vi "DAQmx Read Strain (SubVI).vi"(0 "cDAQ Chassis":i32=2, 5 "9237 (A) Slot":i32=1, 7 "9237 (B) Slot":i32=2, 9 "9237 (C) Slot":i32=2, 11 "Strain Config":T1={"Filter"={"Low-Pass Cut-Off [Hz]"=2.0, "HI/LO Trim [%]"=5.0, "Smooth Size"=3}, "Number of Samples"=6250, "Settings (A)"={"voltage excitation source"=10200, "bridge configuration"=10182, "voltage excitation value"=10.0, "use excitation for scaling"=TRUE, "MIN"=0.0, "MAX"=0.0}, "Settings (B)"={"voltage excitation source"=10200, "bridge configuration"=10182, "voltage excitation value"=10.0, "use excitation for scaling"=TRUE, "MIN"=0.0, "MAX"=0.0}, "Settings (C)"={"voltage excitation source"=10200, "bridge configuration"=10182, "voltage excitation value"=10.0, "use excitation for scaling"=TRUE, "MIN"=0.0, "MAX"=0.0}} {"Settings (C)"."voltage excitation source" items=["Internal"=10200, "External"=10167, "None"=10230]; "Settings (C)"."bridge configuration" items=["Full Bridge"=10182, "Half Bridge"=10187, "Quarter Bridge"=10270, "No Bridge"=10228]; "Settings (B)"."voltage excitation source" items=["Internal"=10200, "External"=10167, "None"=10230]; "Settings (B)"."bridge configuration" items=["Full Bridge"=10182, "Half Bridge"=10187, "Quarter Bridge"=10270, "No Bridge"=10228]; "Settings (A)"."voltage excitation source" items=["Internal"=10200, "External"=10167, "None"=10230]; "Settings (A)"."bridge configuration" items=["Full Bridge"=10182, "Half Bridge"=10187, "Quarter Bridge"=10270, "No Bridge"=10228]}, 12 "Stop Program":bool) -> (4 "Strain Task":refnum<k21>="Relay Control", 6 "(A) Strain":T2 {"Signals" format="%.2p"}, 8 "(B) Strain":T2, 10 "(C) Strain":T2, 13 "Ch0 Raw":dbl[](array[numeric]), 14 "Ch0 Filtered":dbl, 15 "Strain Error":errorcluster={"status"=TRUE, "code"=-200170, "source"="DAQmx Create Channel (DO-Digital Output).vi:1<append>\n<B>Task Name: </B>Relay Control"})   [LabVIEW 2010]
uses:
  <vilib>/Analysis/3filter.llb/Filter Passband Type.ctl
  <vilib>/DAQmx/read.llb/DAQmx Read (Analog 2D DBL NChan NSamp).vi
  <vilib>/daqmx/miscellaneous.llb/DAQmx Fill In Error Info.vi
  <vilib>/Analysis/3filter.llb/Butterworth Filter (DBL).vi
  <vilib>/DAQmx/configure/timing.llb/DAQmx Timing (Sample Clock).vi
  <vilib>/DAQmx/create/channels.llb/DAQmx Create Channel (AI-Voltage-Custom with Excitation).vi
  <vilib>/Analysis/NI_AALBase.lvlib
panel:
  in  "Error Input":errorcluster
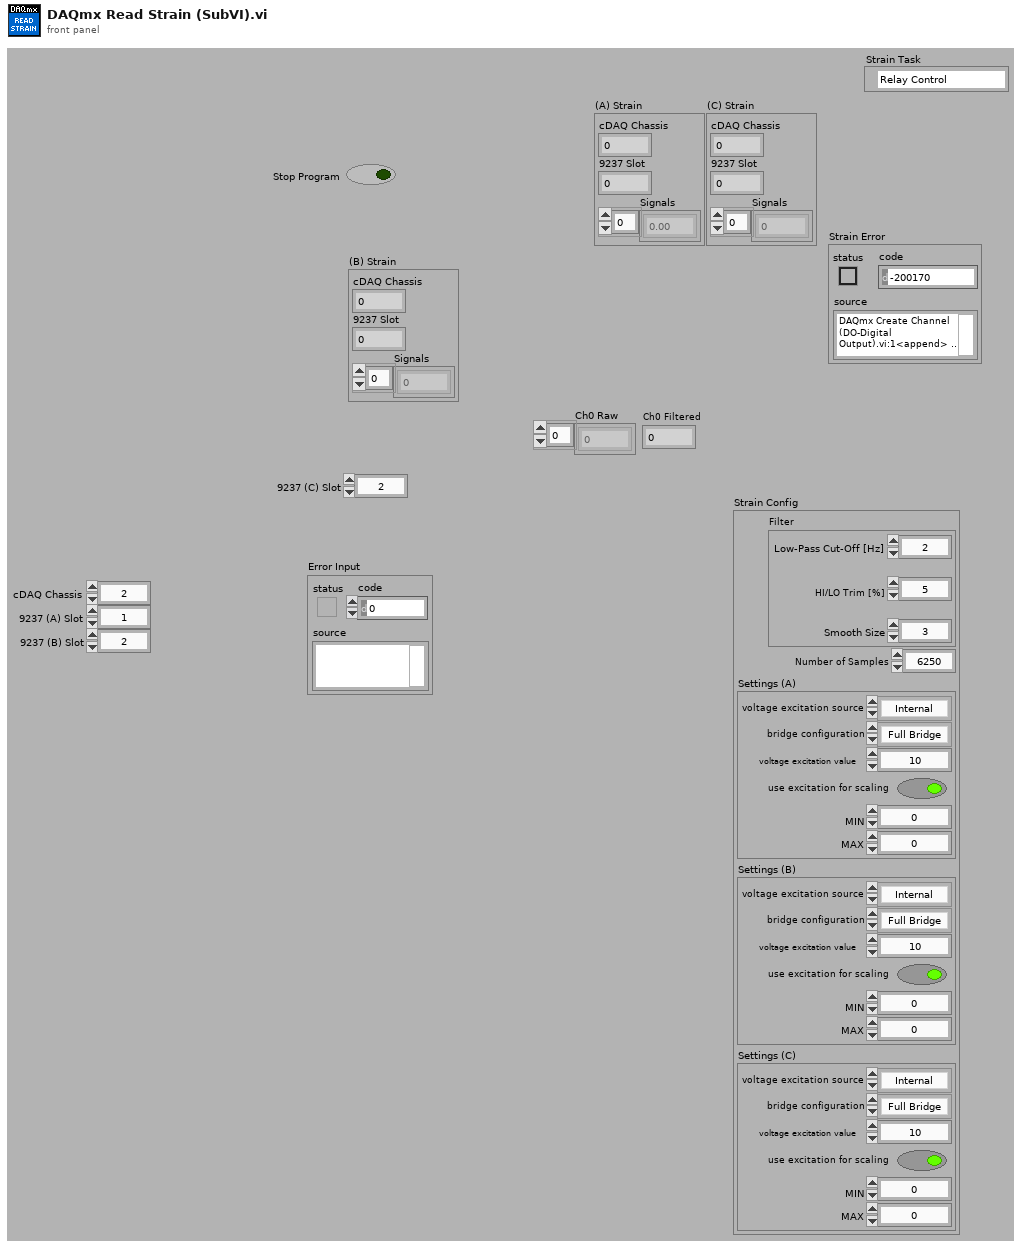
[diagram p1: front panel]
types:
  T1 = cluster{"Filter":cluster{"Low-Pass Cut-Off [Hz]":dbl, "HI/LO Trim [%]":dbl, "Smooth Size":i32}, "Number of Samples":i32, "Settings (A)":cluster{"voltage excitation source":i32, "bridge configuration":i32, "voltage excitation value":dbl, "use excitation for scaling":bool, "MIN":dbl, "MAX":dbl}, "Settings (B)":cluster{"voltage excitation source":i32, "bridge configuration":i32, "voltage excitation value":dbl, "use excitation for scaling":bool, "MIN":dbl, "MAX":dbl}, "Settings (C)":cluster{"voltage excitation source":i32, "bridge configuration":i32, "voltage excitation value":dbl, "use excitation for scaling":bool, "MIN":dbl, "MAX":dbl}}
  T2 = cluster{"cDAQ Chassis":i32, "9237 Slot":i32, "Signals":dbl[]}
  T3 = typedef "NI_AALBase.lvlib/Filter Passband Type.ctl" = enum32{"Lowpass", "Highpass", "Bandpass", "Bandstop"}
  T4 = cluster{"Low-Pass Cut-Off [Hz]":dbl, "HI/LO Trim [%]":dbl, "Smooth Size":i32}
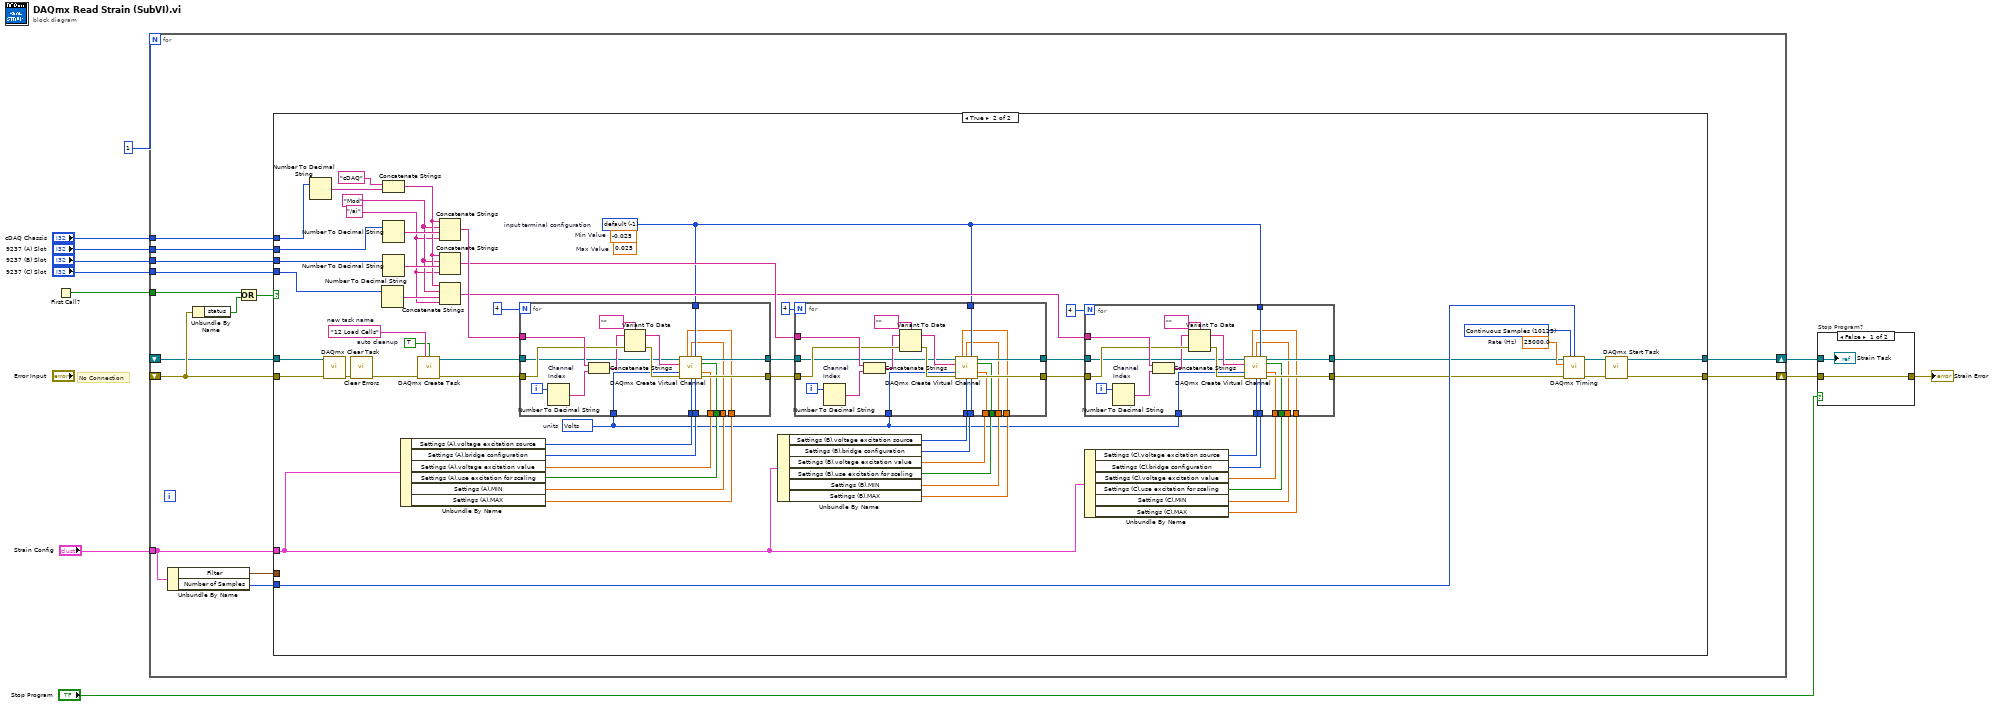
[diagram p0: block diagram]
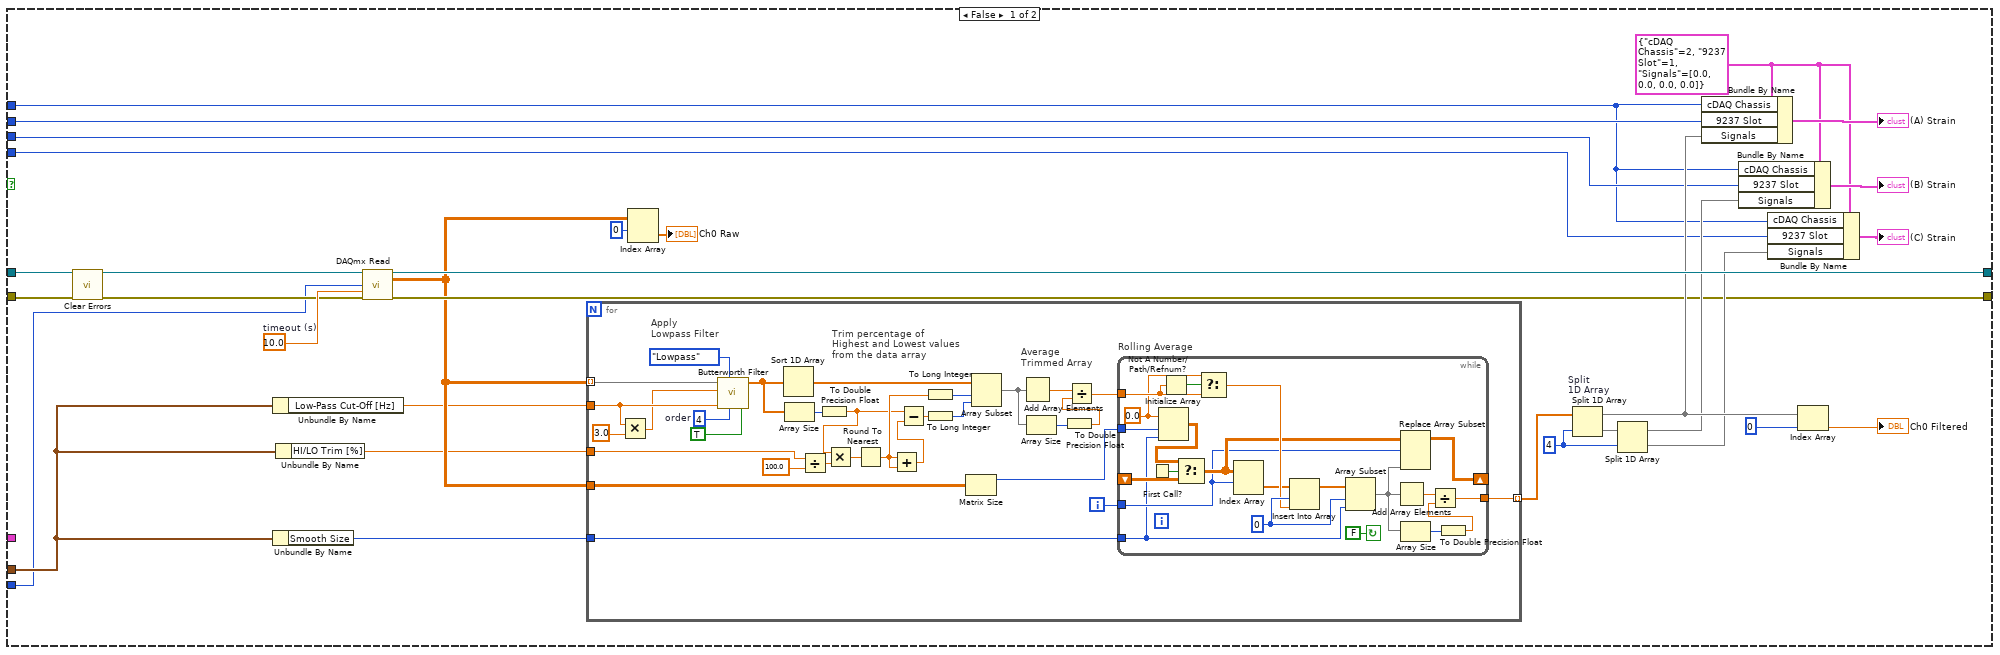
[diagram p2: hidden frame]
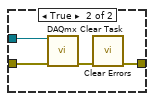
[diagram p3: hidden frame]
diagram:
  # "No Connection"
  n1 = First Call?() -> (First Call?: T/F=w7:bool)
  n2 = for {
    N: 1 -> [_]
    tunnel: "9237 (A) Slot" -> [w25]
    tunnel: "9237 (B) Slot" -> [w24]
    tunnel: "9237 (C) Slot" -> [w23]
    tunnel: "cDAQ Chassis" -> [w22]
    tunnel: w7 -> [w20]
    shift-right: [w18] -> w2
    shift-left: _ -> [w17]
    shift-right: [w16] -> w3
    shift-left: _ -> [w21]
    tunnel: "Strain Config" -> [w12]
    n3 = Unbundle By Name(w12) -> ("Filter"=w14:T4, "Number of Samples"=w13:i32)
    n4 = Unbundle By Name(w21) -> ("status"=w19:bool)
    n5 = Or(x=w20, y=w19) -> (x .or. y?=w15:bool)
    n6 = case shown="True" w15 {
      tunnel: w21 -> [w55 w151]
      tunnel: [w32 w154] -> w16
      tunnel: [w45 w153] -> w18
      tunnel: w17 -> [w46 w152]
      tunnel: w22 -> [w36 w150]
      tunnel: w25 -> [w44 w149]
      tunnel: w24 -> [w40 w148]
      tunnel: w23 -> [w35 w145]
      tunnel: w14 -> [w28 _]
      tunnel: w13 -> [w26 w138]
      tunnel: w12 -> [_ w133]
      frame False {
        w37 = T2 {"cDAQ Chassis"=2, "9237 Slot"=1, "Signals"=[0.0, 0.0, 0.0, 0.0]}
        w49 = 4 ("index")
        w47 = 10.0  # timeout (s)
        n7 = call <vilib>:"Clear Errors.vi"("error in (no error)"=w55) -> ("error out"=w33:errorcluster)  [unwired: 6 in]
        n8 = Unbundle By Name(w28) -> ("Low-Pass Cut-Off [Hz]"=w30:dbl)
        n9 = Unbundle By Name(w28) -> ("Smooth Size"=w27:i32)
        n10 = Unbundle By Name(w28) -> ("HI/LO Trim [%]"=w29:dbl)
        n11 = call-poly <vilib>:"DAQmx Read.vi"("task/channels in"=w46, "number of samples per channel"=w26, "timeout"=w47, "error in"=w33) -> ("task out"=w45:refnum<k21>, "data"=w31:dbl[][], "error out"=w32:errorcluster)  [unwired: 9 in]
        n12 = for {
          tunnel: w31 -> [w82] mode=indexing
          tunnel: [w57] -> w52 mode=indexing
          tunnel: w30 -> [w83]
          tunnel: w31 -> [w60]
          tunnel: w27 -> [w58]
          tunnel: w29 -> [w56]
          i -> [w61]
          w81 = 4  # order
          # "Average\nTrimmed Array"
          # "Trim percentage of\nHighest and Lowest values\nfrom the data array"
          # "Apply \nLowpass Filter"
          n13 = Multiply(x=w83, y=3.0) -> (x*y=w77:dbl)
          n14 = call-poly <vilib>:"Butterworth Filter.vi"("init/cont (init:F)"=TRUE, "order"=w81, "filter type"=Filter_Passband_Type."Lowpass", "low cutoff freq: fl"=w83, "sampling freq: fs"=w77, "X"=w82) -> ("Filtered X"=w85:dbl[])  [unwired: 2 in, 1 out]
          n15 = Sort 1D Array(array=w85) -> (sorted array=w70:dbl[])
          n16 = Array Size(array=w85) -> (size(s)=w76:i32)
          n17 = Divide(x=w56, y=100.0) -> (x/y=w66:dbl)
          n18 = To Double Precision Float(number=w76) -> (double precision float=w68:dbl)
          n19 = Multiply(x=w68, y=w66) -> (x*y=w74:dbl)
          n20 = Round To Nearest(number=w74) -> (nearest integer value=w73:dbl)
          n21 = Add(x=w73, y=w73) -> (x+y=w69:dbl)
          n22 = Subtract(x=w68, y=w69) -> (x-y=w75:dbl)
          n23 = To Long Integer(number=w73) -> (32bit integer=w71:i32)
          n24 = To Long Integer(number=w75) -> (32bit integer=w72:i32)
          n25 = Matrix Size(0:w60) -> (1:w59:i32)  [unwired: 1 out]
          n26 = Array Subset(array=w70, index=w71, length=w72) -> (w84:dbl[])
          n27 = Add Array Elements(numeric array=w84) -> (sum=w64:dbl)
          n28 = Array Size(array=w84) -> (size(s)=w65:i32)
          n29 = To Double Precision Float(number=w65) -> (double precision float=w63:dbl)
          n30 = Divide(x=w64, y=w63) -> (x/y=w62:dbl)
          n31 = while "Rolling Average" {
            tunnel: w62 -> [w104]
            tunnel: w58 -> [w88]
            shift-right: [w94] -> _
            shift-left: _ -> [w92]
            tunnel: [w105] -> w57
            tunnel: w61 -> [w90]
            tunnel: w59 -> [w87]
            stop <- FALSE continue-if-true
            w97 = 0.0
            w102 = 0
            n32 = First Call?() -> (First Call?: T/F=w99:bool)
            n33 = Initialize Array(w97, w87, w88) -> (w89:dbl[][])
            n34 = Not A Number/Path/Refnum?(number/path/refnum=w104) -> (NaN/Path/Refnum?=w98:bool)
            n35 = Select(t=w89, s=w99, f=w92) -> (s? t:f=w91:dbl[][])
            n36 = Select(t=w97, s=w98, f=w104) -> (s? t:f=w96:dbl)
            n37 = Index Array(array=w91, index (row)=w90) -> (element=w93:dbl[])  [unwired: 1 in]
            n38 = Insert Into Array(array=w93, index=w102, new element=w96) -> (w103:dbl[])
            n39 = Array Subset(array=w103, index=w102, length=w88) -> (w95:dbl[])
            n40 = Add Array Elements(numeric array=w95) -> (sum=w101:dbl)
            n41 = Replace Array Subset(array=w91, new element=w95, index (row)=w90) -> (w94:dbl[][])  [unwired: 1 in]
            n42 = Array Size(array=w95) -> (size(s)=w100:i32)
            n43 = To Double Precision Float(number=w100) -> (double precision float=w86:dbl)
            n44 = Divide(x=w101, y=w86) -> (x/y=w105:dbl)
          }
        }
        n45 = Index Array(array=w31, index (row)=0) -> (element=→"Ch0 Raw":dbl[])  [unwired: 1 in]
        n46 = Split 1D Array "Split\n1D Array"(array=w52, index=w49) -> (first subarray=w43:dbl[], second subarray=w48:dbl[])
        n47 = Split 1D Array(array=w48, index=w49) -> (first subarray=w39:dbl[], second subarray=w34:dbl[])
        n48 = Bundle By Name(cluster=w37, "cDAQ Chassis"=w36, "9237 Slot"=w44, "Signals"=w43) -> (→"(A) Strain":T2)
        n49 = Bundle By Name(cluster=w37, "cDAQ Chassis"=w36, "9237 Slot"=w40, "Signals"=w39) -> (→"(B) Strain":T2)
        n50 = Bundle By Name(cluster=w37, "cDAQ Chassis"=w36, "9237 Slot"=w35, "Signals"=w34) -> (→"(C) Strain":T2)
        n51 = Index Array(array=w43, index=0) -> (element=→"Ch0 Filtered":dbl)
      }
      frame True {
        (unwired) 0.025  # Max Value
        (unwired) -0.025  # Min Value
        w139 = 25000.0  # Rate (Hz)
        w140 = 10123 items=["Finite Samples"=10178, "Continuous Samples"=10123, "Hardware Timed Single Point"=12522] ("sample mode")
        w107 = -1 items=["default"=-1, "RSE"=10083, "NRSE"=10078, "Differential"=10106, "Pseudodifferential"=12529]  # input terminal configuration
        w115 = 10348 items=["Volts"=10348, "From Custom Scale"=10065]  # units
        w164 = "12 Load Cells"  # new task name
        w143 = "Mod" ("string")
        w141 = "/ai" ("string")
        w161 = TRUE  # auto cleanup
        n52 = Number To Decimal String(number=w150) -> (decimal integer string=w160:string)  [unwired: 1 in]
        n53 = call <vilib>:"DAQmx Clear Task.vi"("task in"=w152, "error in"=w151) -> ("error out"=w147:errorcluster)  [unwired: 13 in]
        n54 = call <vilib>:"Clear Errors.vi"("error in (no error)"=w147) -> ("error out"=w146:errorcluster)  [unwired: 6 in]
        n55 = Number To Decimal String(number=w145) -> (decimal integer string=w142:string)  [unwired: 1 in]
        n56 = Concatenate Strings("cDAQ" ("string"), w160) -> (w144:string)
        n57 = Number To Decimal String(number=w149) -> (decimal integer string=w158:string)  [unwired: 1 in]
        n58 = Number To Decimal String(number=w148) -> (decimal integer string=w157:string)  [unwired: 1 in]
        n59 = Unbundle By Name(w133) -> ("Settings (A).voltage excitation source"=w137:i32, "Settings (A).bridge configuration"=w134:i32, "Settings (A).voltage excitation value"=w135:dbl, "Settings (A).use excitation for scaling"=w136:bool, "Settings (A).MIN"=w132:dbl, "Settings (A).MAX"=w131:dbl)
        n60 = call <vilib>:"DAQmx Create Task.vi"("new task name"=w164, "auto cleanup"=w161, "error in"=w146) -> ("task out"=w166:refnum<k21>, "error out"=w165:errorcluster)  [unwired: 11 in]
        n61 = Concatenate Strings(w144, w143, w158, w141) -> (w162:string)
        n62 = Concatenate Strings(w144, w143, w157, w141) -> (w130:string)
        n63 = Concatenate Strings(w144, w143, w142, w141) -> (w119:string)
        n64 = for {
          N: 4 -> [_]
          tunnel: w162 -> [w221]
          tunnel: w165 -> [w219]
          tunnel: [w213] -> w127
          tunnel: w166 -> [w215]
          tunnel: [w214] -> w129
          tunnel: w115 -> [w212]
          tunnel: w137 -> [w211]
          tunnel: w134 -> [w210]
          tunnel: w135 -> [w209]
          tunnel: w136 -> [w208]
          tunnel: w107 -> [w207]
          tunnel: w132 -> [w206]
          tunnel: w131 -> [w205]
          i -> [w222]
          n65 = Number To Decimal String "Channel\nIndex"(number=w222) -> (decimal integer string=w223:string)  [unwired: 1 in]
          n66 = Concatenate Strings(w221, w223) -> (w216:string)
          n67 = Variant To Data(error in=w219, Variant=w216, type=tag "" ("physical channels")) -> (error out=w218:errorcluster, data=w217:tag)
          n68 = call-poly <vilib>:"DAQmx Create Virtual Channel.vi"("task in"=w215, "maximum value"=w205, "minimum value"=w206, "input terminal configuration"=w207, "physical channels"=w217, "use excitation for scaling"=w208, "units"=w212, "voltage excitation value"=w209, "error in"=w218, "voltage excitation source"=w211, "bridge configuration"=w210) -> ("task out"=w214:refnum<k21>, "error out"=w213:errorcluster)  [unwired: 3 in]
        }
        n69 = Unbundle By Name(w133) -> ("Settings (B).voltage excitation source"=w126:i32, "Settings (B).bridge configuration"=w125:i32, "Settings (B).voltage excitation value"=w124:dbl, "Settings (B).use excitation for scaling"=w123:bool, "Settings (B).MIN"=w122:dbl, "Settings (B).MAX"=w121:dbl)
        n70 = for {
          N: 4 -> [_]
          tunnel: w130 -> [w202]
          tunnel: w127 -> [w200]
          tunnel: [w194] -> w117
          tunnel: w129 -> [w196]
          tunnel: [w195] -> w118
          tunnel: w115 -> [w193]
          tunnel: w126 -> [w192]
          tunnel: w125 -> [w191]
          tunnel: w124 -> [w190]
          tunnel: w123 -> [w189]
          tunnel: w107 -> [w188]
          tunnel: w122 -> [w187]
          tunnel: w121 -> [w186]
          i -> [w203]
          n71 = Number To Decimal String "Channel\nIndex"(number=w203) -> (decimal integer string=w204:string)  [unwired: 1 in]
          n72 = Concatenate Strings(w202, w204) -> (w197:string)
          n73 = Variant To Data(error in=w200, Variant=w197, type=tag "" ("physical channels")) -> (error out=w199:errorcluster, data=w198:tag)
          n74 = call-poly <vilib>:"DAQmx Create Virtual Channel.vi"("task in"=w196, "maximum value"=w186, "minimum value"=w187, "input terminal configuration"=w188, "physical channels"=w198, "use excitation for scaling"=w189, "units"=w193, "voltage excitation value"=w190, "error in"=w199, "voltage excitation source"=w192, "bridge configuration"=w191) -> ("task out"=w195:refnum<k21>, "error out"=w194:errorcluster)  [unwired: 3 in]
        }
        n75 = Unbundle By Name(w133) -> ("Settings (C).voltage excitation source"=w116:i32, "Settings (C).bridge configuration"=w110:i32, "Settings (C).voltage excitation value"=w111:dbl, "Settings (C).use excitation for scaling"=w112:bool, "Settings (C).MIN"=w113:dbl, "Settings (C).MAX"=w114:dbl)
        n76 = for {
          N: 4 -> [_]
          tunnel: w119 -> [w183]
          tunnel: w117 -> [w181]
          tunnel: [w175] -> w108
          tunnel: w118 -> [w177]
          tunnel: [w176] -> w109
          tunnel: w115 -> [w174]
          tunnel: w116 -> [w173]
          tunnel: w110 -> [w172]
          tunnel: w111 -> [w171]
          tunnel: w112 -> [w170]
          tunnel: w107 -> [w169]
          tunnel: w113 -> [w168]
          tunnel: w114 -> [w167]
          i -> [w184]
          n77 = Number To Decimal String "Channel\nIndex"(number=w184) -> (decimal integer string=w185:string)  [unwired: 1 in]
          n78 = Concatenate Strings(w183, w185) -> (w178:string)
          n79 = Variant To Data(error in=w181, Variant=w178, type=tag "" ("physical channels")) -> (error out=w180:errorcluster, data=w179:tag)
          n80 = call-poly <vilib>:"DAQmx Create Virtual Channel.vi"("task in"=w177, "maximum value"=w167, "minimum value"=w168, "input terminal configuration"=w169, "physical channels"=w179, "use excitation for scaling"=w170, "units"=w174, "voltage excitation value"=w171, "error in"=w180, "voltage excitation source"=w173, "bridge configuration"=w172) -> ("task out"=w176:refnum<k21>, "error out"=w175:errorcluster)  [unwired: 3 in]
        }
        n81 = call-poly <vilib>:"DAQmx Timing.vi"("task/channels in"=w109, "sample mode"=w140, "samples per channel"=w138, "rate"=w139, "error in"=w108) -> ("task out"=w155:refnum<k21>, "error out"=w156:errorcluster)  [unwired: 9 in]
        n82 = call <vilib>:"DAQmx Start Task.vi"("task/channels in"=w155, "error in"=w156) -> ("task out"=w153:refnum<k21>, "error out"=w154:errorcluster)  [unwired: 12 in]
      }
    }
  }
  n83 = case "Stop Program?" shown="False" "Stop Program" {
    tunnel: w2 -> [w225 w227]
    tunnel: w3 -> [w224 w228]
    tunnel: [w224 w226] -> w6
    frame False {
      "Strain Task" <- w225
    }
    frame True {
      n84 = call <vilib>:"DAQmx Clear Task.vi"("task in"=w227, "error in"=w228) -> ("error out"=w229:errorcluster)  [unwired: 13 in]
      n85 = call <vilib>:"Clear Errors.vi"("error in (no error)"=w229) -> ("error out"=w226:errorcluster)  [unwired: 6 in]
    }
  }
  "Strain Error" <- w6
